vi "build.flow-to-inst.delay.vi"(8 "error in":errorcluster, 9 "format string":string, 11 "Step in":variant) -> (0 "error out":errorcluster, 3 "Array":variant[](array[variant]))   [LabVIEW 2024]
uses:
  controls/type.StepFunction.ctl
  Polymorphics/variantCtrlStepFunction.vi
  Polymorphics/variantCtrlSetpoint.vi
  proc.util.validateParamExist.vi
  proc.util.enumToStrStepVar.vi
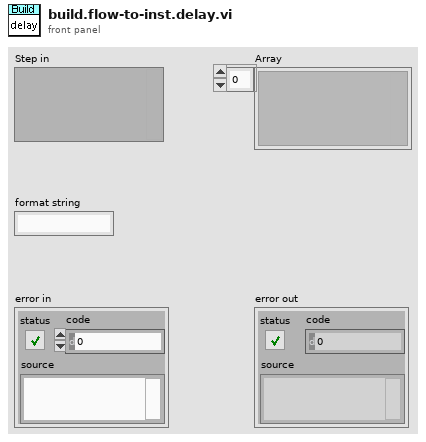
[diagram p1: front panel]
types:
  T1 = typedef "type.StepFunction.ctl" = enum16{"__NO-OP", "_DELAY_LOAD", "_DELAY_COMPARE", "_JUMP", "_COMPLETE", "_COMPARE", "_LOG_MESSAGE", "_LOG_LAST_REPORT", "_SCHEDULE", "_SCHED_DAILY", "CLK_COMPARE", "PROC_START", "PROC_STOP", "PROC_LOAD", "PROC_COMPLETION_CHECK", "PROC_COMPLETION_LOAD", "_IO_READ", "_IO_READ_MANY", "_IO_WRITE", "_IO_WRITE_BY_REG", "_IO_GET_OUTPUT", "_OCS_CHECK", "_OCS_RECORD", "_GET_RH", "_GET_ACC_UV", "_GET_WD", "_GET_WS", "_REC_DELETE", "_REC_MOVE", "_REC_COPY", "_IRR_CHECK", "UNIT_CHECK", "UNIT_SAMPLE", "UNIT_DOSE"}
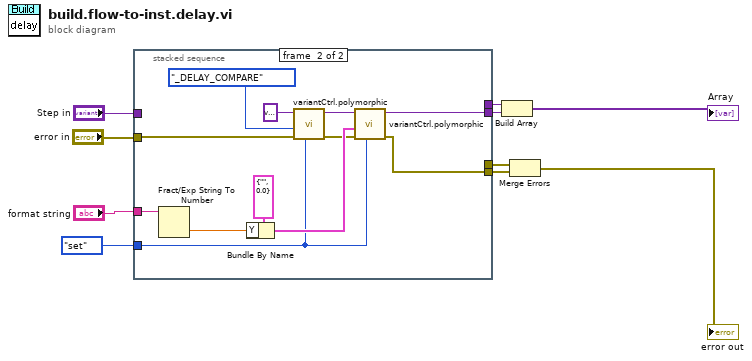
[diagram p0: block diagram]
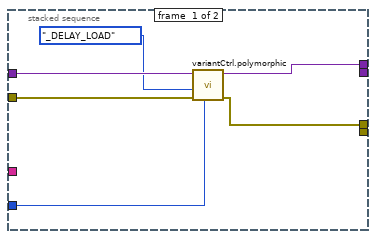
[diagram p2: hidden frame]
diagram:
  n1 = stacked-sequence {
    tunnel: [w14 _] -> w2
    tunnel: [_ w19] -> w3
    tunnel: [_ w27] -> w4
    tunnel: [w13 _] -> w5
    tunnel: "format string" -> [_ w26]
    tunnel: "Step in" -> [w16 _]
    tunnel: enum16{"get", "set"}."set" ("get/set") -> [w15 w22]
    tunnel: "error in" -> [w11 w17]
    frame #0 {
      n2 = call-poly "variantCtrl.polymorphic.vi"("menu in (get)"=w15, "error in"=w11, "StepFunction"=type.StepFunction."_DELAY_LOAD" ("Operation out"), "variant in"=w16) -> ("error out"=w13:errorcluster, "variant out"=w14:variant)  [unwired: 4 in, 2 out]
    }
    frame #1 {
      n3 = Fract/Exp String To Number(string=w26) -> (number=w25:dbl)  [unwired: 3 in, 1 out]
      n4 = Bundle By Name(cluster=cluster{"comparison":string, "Y":dbl} {"comparison"="", "Y"=0.0} ("setpoint 2"), "Y"=w25) -> (w28:cluster{"comparison":string, "Y":dbl})
      n5 = call-poly "variantCtrl.polymorphic.vi"("menu in (get)"=w22, "error in"=w17, "StepFunction"=type.StepFunction."_DELAY_COMPARE" ("Operation out"), "variant in"=variant ("stepElement _DELAY_LOAD")) -> ("error out"=w23:errorcluster, "variant out"=w24:variant)  [unwired: 4 in, 2 out]
      n6 = call-poly "variantCtrl.polymorphic.vi"("get/set"=w22, "error in"=w23, "setpoint"=w28, "procElement in in"=w24) -> ("error out"=w27:errorcluster, "procElement out"=w19:variant)  [unwired: 4 in, 2 out]
    }
  }
  n7 = Build Array(w2, w3) -> (→"Array":variant[])
  n8 = Merge Errors(w5, w4) -> (→"error out":errorcluster)
